vi "Q8381 LEVEL SCALE_LIN-LOG.vi"(1 "off/on":u16(ring) items=["OFF (LOG)", "ON (LINEAR)"], 2 "VISA resource name":refnum<visa-resource-name>, 3 "GPIB Address":u16=8 max=31 step=1) -> (0 "GPIB Status":bool)   [LabVIEW 2017]
doc: "off/on: 0: off(LOG), 1: on(Linear)."
panel:
  out "Programe Code":string
  # "Level scael LIN/LOG"
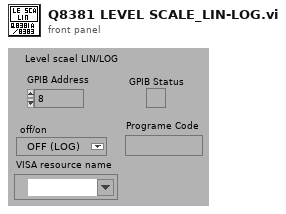
[diagram p1: front panel]
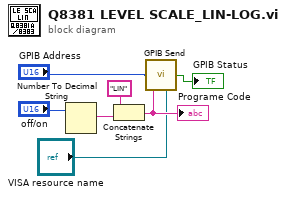
[diagram p0: block diagram]
diagram:
  n1 = Number To Decimal String(number="off/on") -> (decimal integer string=w6:string)  [unwired: 1 in]
  n2 = Concatenate Strings("LIN", w6) -> (w4:string)
  "Programe Code" <- w4
  n3 = call "GPIB Send.vi"("Command String"=w4, "Address"="GPIB Address", "VISA resource name"="VISA resource name") -> ("Error"=→"GPIB Status":bool)
